vi "instr.RelayBD_V02.vi"(6 "测试日志信息":refnum<queue>, 7 "HardWare":enum16{"RelayBD-A", "RelayBD-B", "MCUBD"}(ring), 8 "error in (no error)":errorcluster caption="错误输入（无错误）", 9 "ON/OFF":bool, 10 "Relays":T1(ring), 11 "VISA resource name":refnum<visa-resource-name>="COM1" caption="VISA资源名称") -> (0 "error out":errorcluster caption="错误输出", 3 "OK?":bool)   [LabVIEW 2012, in "Lib_UEL.ATE.lvlib" / "Lib_Instrument.lvlib"]
uses:
  Lib_Instrument.lvlib
  <vilib>/Instr/_visa.llb/VISA Configure Serial Port (Instr).vi
  App/Lib_App.lvlib
panel:
  out "发送字符串":string
  out "返回字符串":string
  out "Return":u8[](array[numeric]) format="%02x"
  in  "timeout (10sec)":u32=1000 caption="超时（10秒）"
  in  "baud rate (9600)":u32=9600 caption="波特率(9600)"
  # "2012-04-17: 确认RelayBD V02可正确工作."
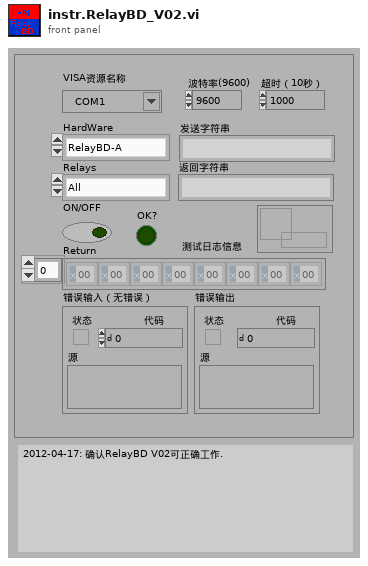
[diagram p1: front panel]
types:
  T1 = enum16{"All", "Group.A", "Group.B", "Relay.A1", "Relay.A2", "Relay.A3", "Relay.A4", "Relay.A5", "Relay.A6", "Relay.A7(BIG)", "Relay.B1", "Relay.B2", "Relay.B3", "Relay.B4", "Relay.B5", "Relay.B6", "Relay.B7(out)", "Check Ver"}
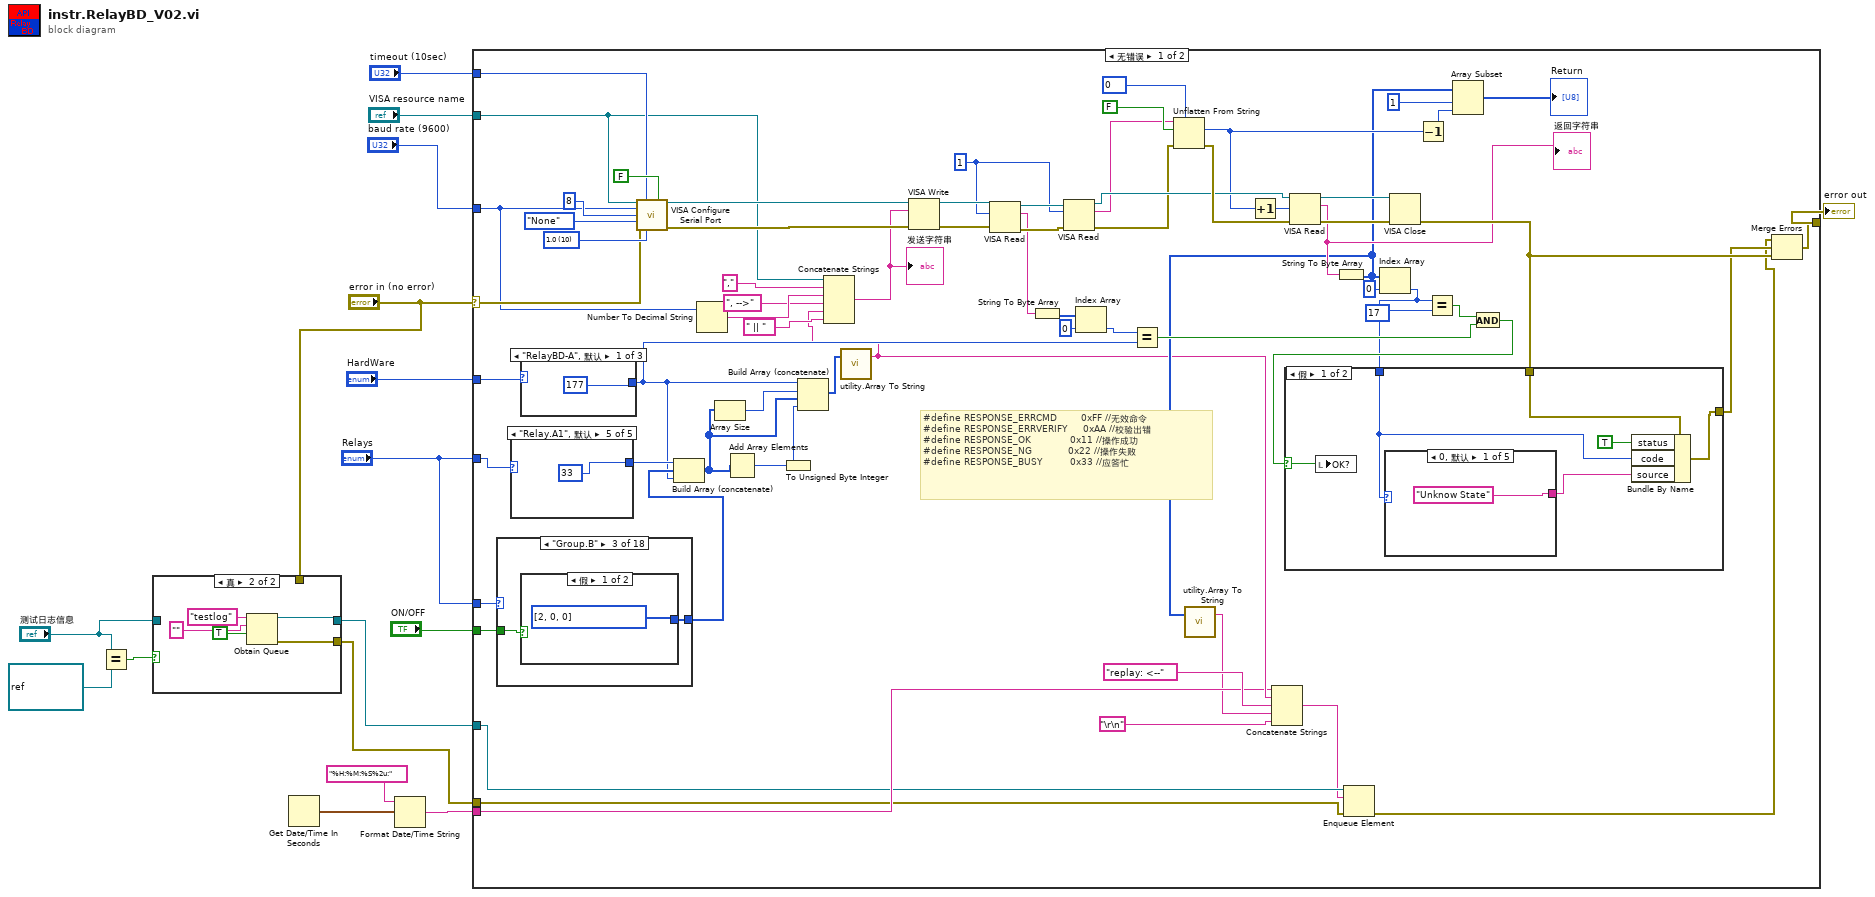
[diagram p0: block diagram]
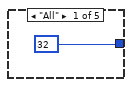
[diagram p3: hidden frame]
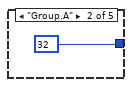
[diagram p4: hidden frame]
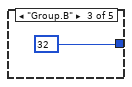
[diagram p5: hidden frame]
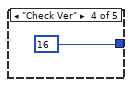
[diagram p6: hidden frame]
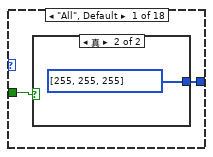
[diagram p7: hidden frame]
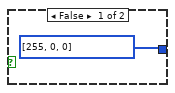
[diagram p8: hidden frame]
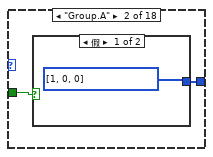
[diagram p9: hidden frame]
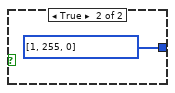
[diagram p10: hidden frame]
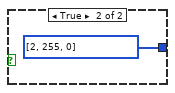
[diagram p11: hidden frame]
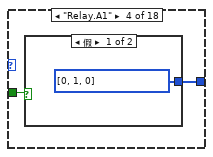
[diagram p12: hidden frame]
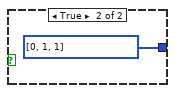
[diagram p13: hidden frame]
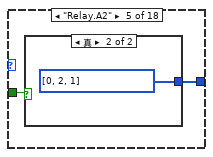
[diagram p14: hidden frame]
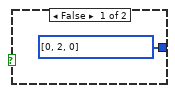
[diagram p15: hidden frame]
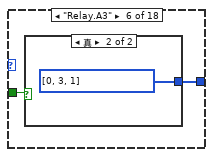
[diagram p16: hidden frame]
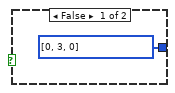
[diagram p17: hidden frame]
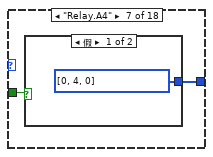
[diagram p18: hidden frame]
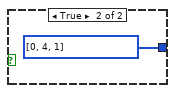
[diagram p19: hidden frame]
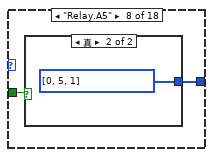
[diagram p20: hidden frame]
diagram:
  n1 = Equal?(x="测试日志信息", y=refnum<queue> refnum) -> (x = y?=w5:bool)
  n2 = case shown="真" w5 {
    tunnel: "测试日志信息" -> [w18 _]
    tunnel: [w18 w23] -> w3
    tunnel: [w17 w22] -> w2
    tunnel: "error in (no error)" -> [w17 _]
    frame False {
    }
    frame True {
      n3 = Obtain Queue(name (unnamed)="testlog" ("名称（未命名）"), element data type="" ("名称（未命名）"), create if not found? (T)=TRUE ("如未找到是否创建？(T)")) -> (queue out=w23:refnum<queue>, error out=w22:errorcluster)  [unwired: 2 in, 1 out]
    }
  }
  n4 = Get Date/Time In Seconds() -> (seconds since 1Jan1904=w8:timestamp)
  n5 = Format Date/Time String(time format string (%c)="%H:%M:%S%2u:" ("时间格式化字符串(%c)"), seconds (now)=w8) -> (date/time string=w7:string)  [unwired: 1 in]
  n6 = case shown="无错误" "error in (no error)" {
    selector: "error in (no error)" -> [w79 w184]
    tunnel: "VISA resource name" -> [w36 _]
    tunnel: [w45 w183] -> w12
    tunnel: "baud rate (9600)" -> [w37 _]
    tunnel: "timeout (10sec)" -> [w86 _]
    tunnel: "HardWare" -> [w78 _]
    tunnel: "Relays" -> [w52 _]
    tunnel: "Relays" -> [w56 _]
    tunnel: "ON/OFF" -> [w55 _]
    tunnel: w3 -> [w27 w187]
    tunnel: w7 -> [w29 w186]
    tunnel: w2 -> [w26 _]
    frame No Error {
      w84 = u16 10 items=["1.0"=10, "1.5"=15, "2.0"=20] ("stop bits (10: 1 bit)")
      w70 = u32 1 ("字节总数")
      # "#define RESPONSE_ERRCMD     \t\t\t0xFF\t//无效命令 \n#define RESPONSE_ERRVERIFY\t\t\t  0xAA\t//校验出错 \n#define RESPONSE_OK           \t\t0x11\t//操作成功 \n#define RESPONSE_NG         \t\t\t0x22\t//操作失败 \n#define RESPONSE_BUSY     \t\t\t\t0x33\t//应答忙"
      n7 = case shown="\"Group.B\"" w56 {
        tunnel: w55 -> [w99 w103 w107 w111 w115 w119 w123 w127 w131 w135 w139 w143 w147 w151 w155 w159 w163 _]
        tunnel: [w98 w102 w106 w110 w114 w118 w122 w126 w130 w134 w138 w142 w146 w150 w154 w158 w162 u8[] [] ("数组")] -> w54
        frame "All", Default {
          n8 = case shown="真" w99 {
            tunnel: [u8[] [255, 0, 0] ("数组") u8[] [255, 255, 255] ("数组")] -> w98
            frame False {
            }
            frame True {
            }
          }
        }
        frame "Group.A" {
          n9 = case shown="假" w103 {
            tunnel: [u8[] [1, 0, 0] ("数组") u8[] [1, 255, 0] ("数组")] -> w102
            frame False {
            }
            frame True {
            }
          }
        }
        frame "Group.B" {
          n10 = case shown="假" w107 {
            tunnel: [u8[] [2, 0, 0] ("数组") u8[] [2, 255, 0] ("数组")] -> w106
            frame False {
            }
            frame True {
            }
          }
        }
        frame "Relay.A1" {
          n11 = case shown="假" w111 {
            tunnel: [u8[] [0, 1, 0] ("数组") u8[] [0, 1, 1] ("数组")] -> w110
            frame False {
            }
            frame True {
            }
          }
        }
        frame "Relay.A2" {
          n12 = case shown="真" w115 {
            tunnel: [u8[] [0, 2, 0] ("数组") u8[] [0, 2, 1] ("数组")] -> w114
            frame False {
            }
            frame True {
            }
          }
        }
        frame "Relay.A3" {
          n13 = case shown="真" w119 {
            tunnel: [u8[] [0, 3, 0] ("数组") u8[] [0, 3, 1] ("数组")] -> w118
            frame False {
            }
            frame True {
            }
          }
        }
        frame "Relay.A4" {
          n14 = case shown="假" w123 {
            tunnel: [u8[] [0, 4, 0] ("数组") u8[] [0, 4, 1] ("数组")] -> w122
            frame False {
            }
            frame True {
            }
          }
        }
        frame "Relay.A5" {
          n15 = case shown="真" w127 {
            tunnel: [u8[] [0, 5, 0] ("数组") u8[] [0, 5, 1] ("数组")] -> w126
            frame False {
            }
            frame True {
            }
          }
        }
        frame "Relay.A6" {
          n16 = case shown="假" w131 {
            tunnel: [u8[] [0, 6, 0] ("数组") u8[] [0, 6, 1] ("数组")] -> w130
            frame False {
            }
            frame True {
            }
          }
        }
        frame "Relay.A7(BIG)" {
          n17 = case shown="真" w135 {
            tunnel: [u8[] [0, 7, 0] ("数组") u8[] [0, 7, 1] ("数组")] -> w134
            frame False {
            }
            frame True {
            }
          }
        }
        frame "Relay.B1" {
          n18 = case shown="真" w139 {
            tunnel: [u8[] [1, 1, 0] ("数组") u8[] [1, 1, 1] ("数组")] -> w138
            frame False {
            }
            frame True {
            }
          }
        }
        frame "Relay.B2" {
          n19 = case shown="假" w143 {
            tunnel: [u8[] [1, 2, 0] ("数组") u8[] [1, 2, 1] ("数组")] -> w142
            frame False {
            }
            frame True {
            }
          }
        }
        frame "Relay.B3" {
          n20 = case shown="真" w147 {
            tunnel: [u8[] [1, 3, 0] ("数组") u8[] [1, 3, 1] ("数组")] -> w146
            frame False {
            }
            frame True {
            }
          }
        }
        frame "Relay.B4" {
          n21 = case shown="假" w151 {
            tunnel: [u8[] [1, 4, 0] ("数组") u8[] [1, 4, 1] ("数组")] -> w150
            frame False {
            }
            frame True {
            }
          }
        }
        frame "Relay.B5" {
          n22 = case shown="真" w155 {
            tunnel: [u8[] [1, 5, 0] ("数组") u8[] [1, 5, 1] ("数组")] -> w154
            frame False {
            }
            frame True {
            }
          }
        }
        frame "Relay.B6" {
          n23 = case shown="假" w159 {
            tunnel: [u8[] [1, 6, 0] ("数组") u8[] [1, 6, 1] ("数组")] -> w158
            frame False {
            }
            frame True {
            }
          }
        }
        frame "Relay.B7(out)" {
          n24 = case shown="真" w163 {
            tunnel: [u8[] [1, 7, 0] ("数组") u8[] [1, 7, 1] ("数组")] -> w162
            frame False {
            }
            frame True {
            }
          }
        }
        frame "Check Ver" {
        }
      }
      n25 = case shown="\"Relay.A1\", 默认" w52 {
        tunnel: [u8 32 u8 32 u8 32 u8 16 u8 33] -> w51
        frame "All" {
        }
        frame "Group.A" {
        }
        frame "Group.B" {
        }
        frame "Check Ver" {
        }
        frame "Relay.A1", Default {
        }
      }
      n26 = case shown="\"RelayBD-A\", 默认" w78 {
        tunnel: [u8 177 u8 178 u8 161] -> w42
        frame "RelayBD-A", Default {
        }
        frame "RelayBD-B" {
        }
        frame "MCUBD" {
        }
      }
      n27 = call-poly "VISA Configure Serial Port"("VISA resource name"=w36, "timeout (10sec)"=w86, "Enable Termination\nChar (T)"=FALSE ("Enable Termination\nChar (T)"), "baud rate (9600)"=w37, "data bits (8)"=u16 8, "parity (0:none)"=enum16{"None", "Odd", "Even", "Mark", "Space"}."None", "error in (no error)"=w79, "stop bits (10: 1 bit)"=w84) -> ("VISA resource name out"=w83:refnum<visa-resource-name>, "error out"=w74:errorcluster)  [unwired: 6 in]
      n28 = Build Array (concatenate)(w51, w54, w42) -> (w76:u8[])
      n29 = Number To Decimal String(number=w37) -> (decimal integer string=w41:string)  [unwired: 1 in]
      n30 = Array Size(array=w76) -> (size(s)=w77:i32)
      n31 = Add Array Elements(numeric array=w76) -> (sum=w44:u8)
      n32 = To Unsigned Byte Integer(number=w44) -> (unsigned 8bit integer=w75:u8)
      n33 = Build Array (concatenate)(w42, w77, w76, w75) -> (w35:i32[])
      n34 = call "utility.Array To String.vi"("无符号字节数组"=w35) -> ("命令输出(字符串)"=w30:string)  [unwired: 1 in, 1 out]
      n35 = Concatenate Strings(w36, "," ("字符串"), w41, ", -->" ("字符串"), w30, " || " ("字符串")) -> (w31:string)
      "发送字符串" <- w31
      n36 = VISA Write(VISA resource name=w83, write buffer=w31, error in (no error)=w74) -> (VISA resource name out=w91:refnum<visa-resource-name>, error out=w90:errorcluster)  [unwired: 1 out]
      n37 = VISA Read(VISA resource name=w91, byte count=w70, error in (no error)=w90) -> (VISA resource name out=w71:refnum<visa-resource-name>, read buffer=w66:string, error out=w72:errorcluster)  [unwired: 1 out]
      n38 = String To Byte Array(string=w66) -> (unsigned byte array=w65:u8[])
      n39 = VISA Read(VISA resource name=w71, byte count=w70, error in (no error)=w72) -> (VISA resource name out=w69:refnum<visa-resource-name>, read buffer=w67:string, error out=w68:errorcluster)  [unwired: 1 out]
      n40 = Index Array(array=w65, index=0 ("索引")) -> (element=w63:u8)
      n41 = Equal?(x=w63, y=w42) -> (x = y?=w59:bool)
      n42 = Unflatten From String(type=u8 0, binary string=w67, data includes array or string size? (T)=FALSE ("数据中包含数组或字符串大小？(T)"), error in (no error)=w68) -> (value=w48:u8, error out=w80:errorcluster)  [unwired: 1 in, 1 out]
      n43 = Increment(x=w48) -> (x+1=w73:u8)
      n44 = VISA Read(VISA resource name=w69, byte count=w73, error in (no error)=w80) -> (VISA resource name out=w89:refnum<visa-resource-name>, read buffer=w43:string, error out=w88:errorcluster)  [unwired: 1 out]
      "返回字符串" <- w43
      n45 = String To Byte Array(string=w43) -> (unsigned byte array=w32:u8[])
      n46 = call "utility.Array To String.vi"("无符号字节数组"=w32) -> ("命令输出(字符串)"=w28:string)  [unwired: 1 in, 1 out]
      n47 = Concatenate Strings(w29, w30, "replay: <--" ("字符串"), w28, "\r\n") -> (w25:string)
      n48 = Enqueue Element(queue=w27, element=w25, error in (no error)=w26) -> (error out=w24:errorcluster)  [unwired: 1 in, 2 out]
      n49 = Index Array(array=w32, index=0 ("索引")) -> (element=w49:u8)
      n50 = VISA Close(VISA resource name=w89, error in (no error)=w88) -> (error out=w47:errorcluster)
      n51 = Decrement(x=w48) -> (x-1=w50:u8)
      n52 = Equal?(x=w49, y=u8 17) -> (x = y?=w60:bool)
      n53 = Array Subset(array=w32, index=1 ("索引"), length=w50) -> (→"Return":u8[])
      n54 = And(x=w60, y=w59) -> (x .and. y?=w58:bool)
      n55 = case shown="假" w58 {
        selector: w58 -> [w172 w179]
        tunnel: [w169 w178] -> w46
        tunnel: w47 -> [w171 w178]
        tunnel: w49 -> [w168 _]
        frame False {
          n56 = local write "OK?"(w172) -> ()
          n57 = case shown="0, 默认" w168 {
            tunnel: ["Unknow State" ("source") "Wrong CMD" ("source") "Verify Err" ("source") "Fail" ("source") "Busy" ("source")] -> w167
            frame 0, Default {
            }
            frame 255 {
            }
            frame 170 {
            }
            frame 34 {
            }
            frame 35 {
            }
          }
          n58 = Bundle By Name(cluster=w171, "status"=TRUE, "code"=w168, "source"=w167) -> (w169:errorcluster)
        }
        frame True {
          "OK?" <- w179
        }
      }
      n59 = Merge Errors(w24, w46, w47) -> (w45:errorcluster)
    }
    frame Error {
      n60 = Concatenate Strings(w186, "ERR Input." ("字符串"), "\r\n") -> (w188:string)
      n61 = Enqueue Element(queue=w187, element=w188, error in (no error)=errorcluster {"status"=FALSE, "code"=0, "source"=""} ("错误输入（无错误）")) -> (error out=w185:errorcluster)  [unwired: 1 in, 2 out]
      n62 = Merge Errors(w184, w185) -> (w183:errorcluster)
      n63 = local write "OK?"(FALSE ("OK?")) -> ()
    }
  }
  "error out" <- w12
